vi "Client.vi"() -> ()   [LabVIEW 2015]
uses:
  <vilib>/Instr/_visa.llb/VISA Configure Serial Port (Instr).vi
panel:
  out "Meter":i32(knob) scale=200.0..255.0
  out "VISA":string
  out "Connection":string
  out "Feedback":string
  out "Command to send":string
  out "Information":string
  out "Error out VISA Read":errorcluster
  in  "baud rate (115200)":u32=115200
  out "Board on port":refnum<visa-resource-name>
  out "Board status":bool
  in  "Board name":string="Arduino"
  out "Error out TCP":errorcluster
  in  "Connect":bool
  in  "Remote port":u16=22022
  out "IP Address of this PC":string
  out "Domain":string
  in  "Stop Sim":bool
  in  "Address IP of remote PC":string
  # "Client"
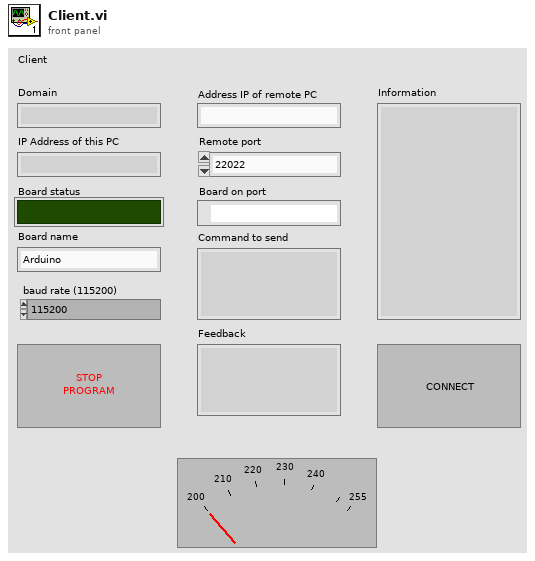
[diagram p1: front panel]
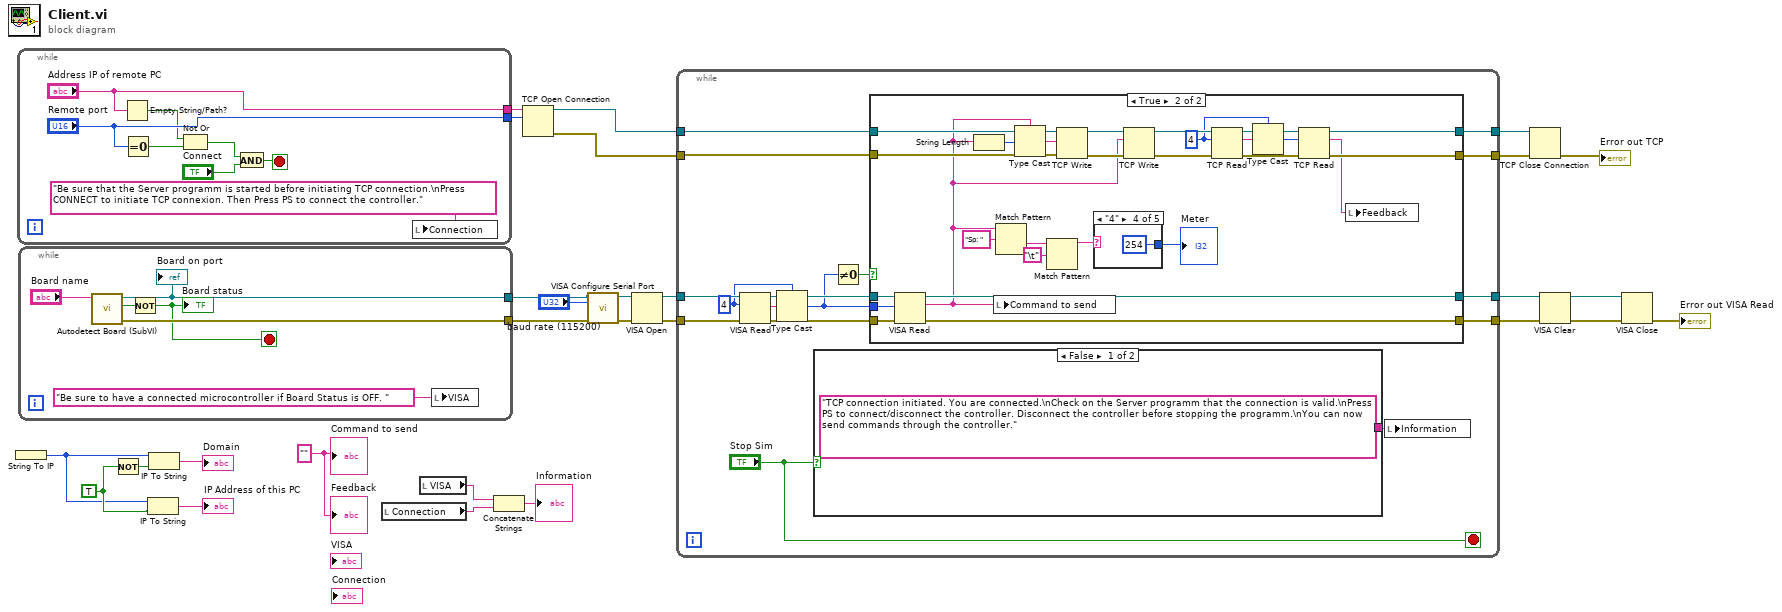
[diagram p0: block diagram]
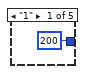
[diagram p3: hidden frame]
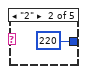
[diagram p4: hidden frame]
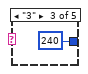
[diagram p5: hidden frame]
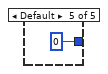
[diagram p6: hidden frame]
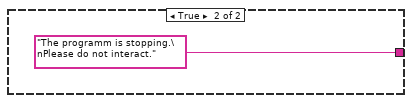
[diagram p7: hidden frame]
diagram:
  w3 = ""
  w19 = TRUE
  n1 = String To IP() -> (0:w18:u32)  [unwired: 1 in]
  n2 = while {
    tunnel: ["Remote port"] -> w28
    tunnel: ["Address IP of remote PC"] -> w27
    stop <- w32 stop-if-true
    n3 = Empty String/Path?(string/path="Address IP of remote PC") -> (empty?=w33:bool)
    n4 = Equal To 0?(x="Remote port") -> (x = 0?=w34:bool)
    n5 = Not Or(1:w34, 2:w33) -> (0:w31:bool)
    n6 = And(x=w31, y="Connect") -> (x .and. y?=w32:bool)
    n7 = local write "Connection"("Be sure that the Server programm is started before initiating TCP connection.\nPress CONNECT to initiate TCP connexion. Then Press PS to connect the controller.") -> ()
  }
  n8 = while {
    tunnel: [w41] -> w17
    tunnel: [w40] -> w16
    stop <- w38 stop-if-true
    n9 = call "Autodetect Board (SubVI).vi"("instr name"="Board name") -> ("error out"=w40:errorcluster, "status"=w39:bool, "VISA Refnum out"=w41:refnum<visa-resource-name>)  [unwired: 8 in]
    "Board on port" <- w41
    n10 = Not(x=w39) -> (.not. x?=w38:bool)
    "Board status" <- w38
    n11 = local write "VISA"("Be sure to have a connected microcontroller if Board Status is OFF. ") -> ()
  }
  n12 = Not(x=w19) -> (.not. x?=w20:bool)
  n13 = IP To String(1:w19, 2:w18) -> (0:→"IP Address of this PC":string)
  n14 = IP To String(1:w20, 2:w18) -> (0:→"Domain":string)
  n15 = local read "Connection"() -> (w1:string)
  n16 = local read "VISA"() -> (w2:string)
  n17 = Concatenate Strings(w2, w1) -> (→"Information":string)
  n18 = TCP Open Connection(address=w27, remote port or service name=w28) -> (connection ID=w26:refnum<k5>, error out=w25:errorcluster)  [unwired: 3 in]
  n19 = call-poly "VISA Configure Serial Port"("VISA resource name"=w17, "baud rate (9600)"="baud rate (115200)", "error in (no error)"=w16) -> ("VISA resource name out"=w14:refnum<visa-resource-name>, "error out"=w13:errorcluster)  [unwired: 11 in]
  n20 = VISA Open(error in (no error)=w13, VISA resource name=w14) -> (VISA resource name=w12:refnum<visa-resource-name>, error out=w11:errorcluster)  [unwired: 3 in]
  n21 = while {
    tunnel: w26 -> [w58]
    tunnel: [w56] -> w24
    tunnel: w25 -> [w57]
    tunnel: [w55] -> w23
    tunnel: w12 -> [w54]
    tunnel: [w46] -> w10
    tunnel: w11 -> [w53]
    tunnel: [w45] -> w9
    stop <- "Stop Sim" stop-if-true
    w48 = u32 4 ("byte count")
    n22 = VISA Read(VISA resource name=w54, byte count=w48, error in (no error)=w53) -> (VISA resource name out=w51:refnum<visa-resource-name>, read buffer=w49:string, error out=w50:errorcluster)  [unwired: 1 out]
    n23 = Type Cast(type=w48, x=w49) -> (*(type *) &x=w43:u32)
    n24 = case shown="False" "Stop Sim" {
      tunnel: ["TCP connection initiated. You are connected.\nCheck on the Server programm that the connection is valid.\nPress PS to connect/disconnect the controller. Disconnect the controller before stopping the programm.\nYou can now send commands through the controller." "The programm is stopping.\nPlease do not interact."] -> w52
      frame False {
      }
      frame True {
      }
    }
    n25 = Not Equal To 0?(x=w43) -> (x != 0?=w44:bool)
    n26 = case shown="True" w44 {
      tunnel: w58 -> [w62 w89]
      tunnel: w57 -> [w61 w88]
      tunnel: [w62 w75] -> w56
      tunnel: [w61 w74] -> w55
      tunnel: w51 -> [w60 w83]
      tunnel: w50 -> [w59 w82]
      tunnel: w43 -> [_ w81]
      tunnel: [w60 w70] -> w46
      tunnel: [w59 w80] -> w45
      frame False {
      }
      frame True {
        w72 = 4
        n27 = VISA Read(VISA resource name=w83, byte count=w81, error in (no error)=w82) -> (VISA resource name out=w70:refnum<visa-resource-name>, read buffer=w69:string, error out=w80:errorcluster)  [unwired: 1 out]
        n28 = String Length(string=w69) -> (length=w85:i32)
        n29 = local write "Command to send"(w69) -> ()
        n30 = Match Pattern(string=w69, regular expression="Sp: ") -> (after substring=w67:string)  [unwired: 1 in, 3 out]
        n31 = Type Cast(type=w69, x=w85) -> (*(type *) &x=w84:string)
        n32 = Match Pattern(string=w67, regular expression="\t") -> (before substring=w64:string)  [unwired: 1 in, 3 out]
        n33 = TCP Write(connection ID=w89, data in=w84, error in (no error)=w88) -> (connection ID out=w87:refnum<k5>, error out=w86:errorcluster)  [unwired: 1 in, 1 out]
        n34 = case shown="\"4\"" w64 {
          tunnel: [200 220 240 254 0] -> w65
          frame "1" {
          }
          frame "2" {
          }
          frame "3" {
          }
          frame "4" {
          }
          frame Default {
          }
        }
        "Meter" <- w65
        n35 = TCP Write(connection ID=w87, data in=w69, error in (no error)=w86) -> (connection ID out=w79:refnum<k5>, error out=w78:errorcluster)  [unwired: 1 in, 1 out]
        n36 = TCP Read(connection ID=w79, bytes to read=w72, error in (no error)=w78) -> (connection ID out=w77:refnum<k5>, data out=w73:string, error out=w76:errorcluster)  [unwired: 2 in]
        n37 = Type Cast(type=w72, x=w73) -> (*(type *) &x=w71:i32)
        n38 = TCP Read(connection ID=w77, bytes to read=w71, error in (no error)=w76) -> (connection ID out=w75:refnum<k5>, data out=w63:string, error out=w74:errorcluster)  [unwired: 2 in]
        n39 = local write "Feedback"(w63) -> ()
      }
    }
    n40 = local write "Information"(w52) -> ()
  }
  n41 = TCP Close Connection(connection ID=w24, error in (no error)=w23) -> (error out=→"Error out TCP":errorcluster)  [unwired: 1 in, 1 out]
  n42 = VISA Clear(VISA resource name=w10, error in (no error)=w9) -> (VISA resource name out=w8:refnum<visa-resource-name>, error out=w7:errorcluster)
  n43 = VISA Close(VISA resource name=w8, error in (no error)=w7) -> (error out=→"Error out VISA Read":errorcluster)
  "Command to send" <- w3
  "Feedback" <- w3
